vi "Dashboard Main.vi"() -> ()   [LabVIEW 2015]
uses:
  <vilib>/Utility/miscctls.llb/LVRowAndColumnTypeDef.ctl
  <vilib>/event_ctls.llb/eventvkey.ctl
  <vilib>/Rock Robotics/WPI/Dashboard/WPI_DashboardLogging Global.vi
  <vilib>/Rock Robotics/Network Tables/NT Read Numeric Array.vi
  <vilib>/Utility/config.llb/Write Key (String).vi
  <vilib>/Utility/config.llb/Write Key (I32).vi
  <vilib>/Utility/config.llb/NI_LVConfig.lvlib
panel:
  in  "Camera Settings 2":T1={"Frame Rate"=30, "Compression"=30, "Size"=1} {"Frame Rate" scale=1.0..30.0; "Size" items=["640x480", "320x240", "160x120"]}
  out "Camera IP 2":string
  in  "Rec Mode 2":enum32{"Stop", "Record", "Playback"}(radio)
  in  "Vision 2":u16(ring) items=["Camera Off", "USB Camera SW", "USB Camera HW", "IP Camera"]
  in  "TCP":refnum<k5>
  in  "Rec Mode":enum32{"Stop", "Record", "Playback"}(radio)
  in  "Vision":u16(ring) items=["Camera Off", "USB Camera SW", "USB Camera HW", "IP Camera"]
  out "Camera IP":string
  out "Image Message":string="Timeout in Camera Communications"
  in  "Dashboard Tab":T2(tab)
  in  "Select Auto":string(combo)
  out "NT Connection":bool
  in  "Camera Settings":T1={"Frame Rate"=30, "Compression"=30, "Size"=1} {"Frame Rate" scale=1.0..30.0; "Size" items=["640x480", "320x240", "160x120"]}
  out "MotorChart R":cluster{"Numeric":dbl, "Numeric":dbl}(graph)
  out "MotorChart L":T3(graph)
  out "MotorSliders R":cluster{"MotorSlide1":dbl, "MotorSlide2":dbl} {"MotorSlide2" scale=-1.0..1.0 scale format="%#_2e"; "MotorSlide1" scale=-1.0..1.0 scale format="%#_2e"}
  out "MotorSliders L":T4 {"MotorSlide4 2" scale=0.0..14.0 scale format="%#_2e"; "MotorSlide2" scale=-1.0..1.0 scale format="%#_2e"; "MotorSlide1" scale=-1.0..1.0 scale format="%#_2e"}
  out "JS1 Z":dbl(slide) scale=-1.0..1.0 scale format="%#_2e"
  out "JS1 Graph":cluster{"X":dbl, "Y":dbl}[](graph)
  out "JS1 Buttons":T5
  out "JS2 Z":dbl(slide) scale=-1.0..1.0 scale format="%#_2e"
  out "JS2 Graph":cluster{"X":dbl, "Y":dbl}[](graph)
  out "JS2 Buttons":T5
  out "Mode":T6(ring)=enum."Auto Disabled"
  in  "DB Camera Config":bool
  out "fps":dbl format="%#.1g"
  out "Mbps":dbl format="%#.1g"
  out "Mbps LED":bool
  out "Camera Image 2":T7(plugin-control)
  out "Mbps 2":dbl format="%#.1g"
  out "fps 2":dbl format="%#.1g"
  in  "DB/String 9":string
  in  "DB/String 8":string
  in  "DB/String 7":string
  in  "DB/String 6":string
  in  "DB/String 5":string
  in  "DB/String 4":string
  in  "DB/String 3":string
  in  "DB/String 2":string
  in  "DB/String 1":string
  in  "DB/String 0":string
  in  "DB/Slider 0":dbl(slide) scale=0.0..5.0
  in  "DB/Slider 1":dbl(slide) scale=0.0..5.0
  in  "DB/Slider 2":dbl(slide) scale=0.0..5.0
  in  "DB/Slider 3":dbl(slide) scale=0.0..5.0
  out "DB/LED 3":bool
  out "DB/LED 2":bool
  out "DB/LED 1":bool
  out "DB/LED 0":bool
  in  "DB/Button 3":bool
  in  "DB/Button 2":bool
  in  "DB/Button 1":bool
  in  "DB/Button 0":bool caption="New Name"
  in  "Test Slider":dbl(slide) scale=0.0..100.0 scale format="%#_3g"
  in  "On/Off":bool caption="Solenoid"
  in  "Test Name":u16(ring) items=["Select the test to run..."]
  in  "Test Tree":string(tree)
  in  "Motor":cluster{"Value":dbl, "Enable":bool} {"Value" scale=-1.0..1.0 scale format="%#_3g"}
  out "Progress":T8 {"Test Progress" scale=0.0..100.0}
  in  "Rev/Fwd":cluster{"Forward":bool, "Reverse":bool}
  in  "Test Ring":u16(ring) items=["Monochrome", "Color"]
  out "Cmd Status":string
  in  "Execute Command":bool
  in  "Command Params":string[][](table)
  in  "Command Selection":i32(listbox)
  in  "CheckList":i32(listbox)
  out "Tree":string(tree)
  out "Camera Image":T7(plugin-control)
  out "Background":bool
  # "Left"
  # "Front"
  # "Right"
  # "Battery"
  # "This tab is a great place for autonomous settings and robot-specific values.\nPlace controls and indicators inside this tab and match name to\nDashboard Variables on robot. You can also delete this comment."
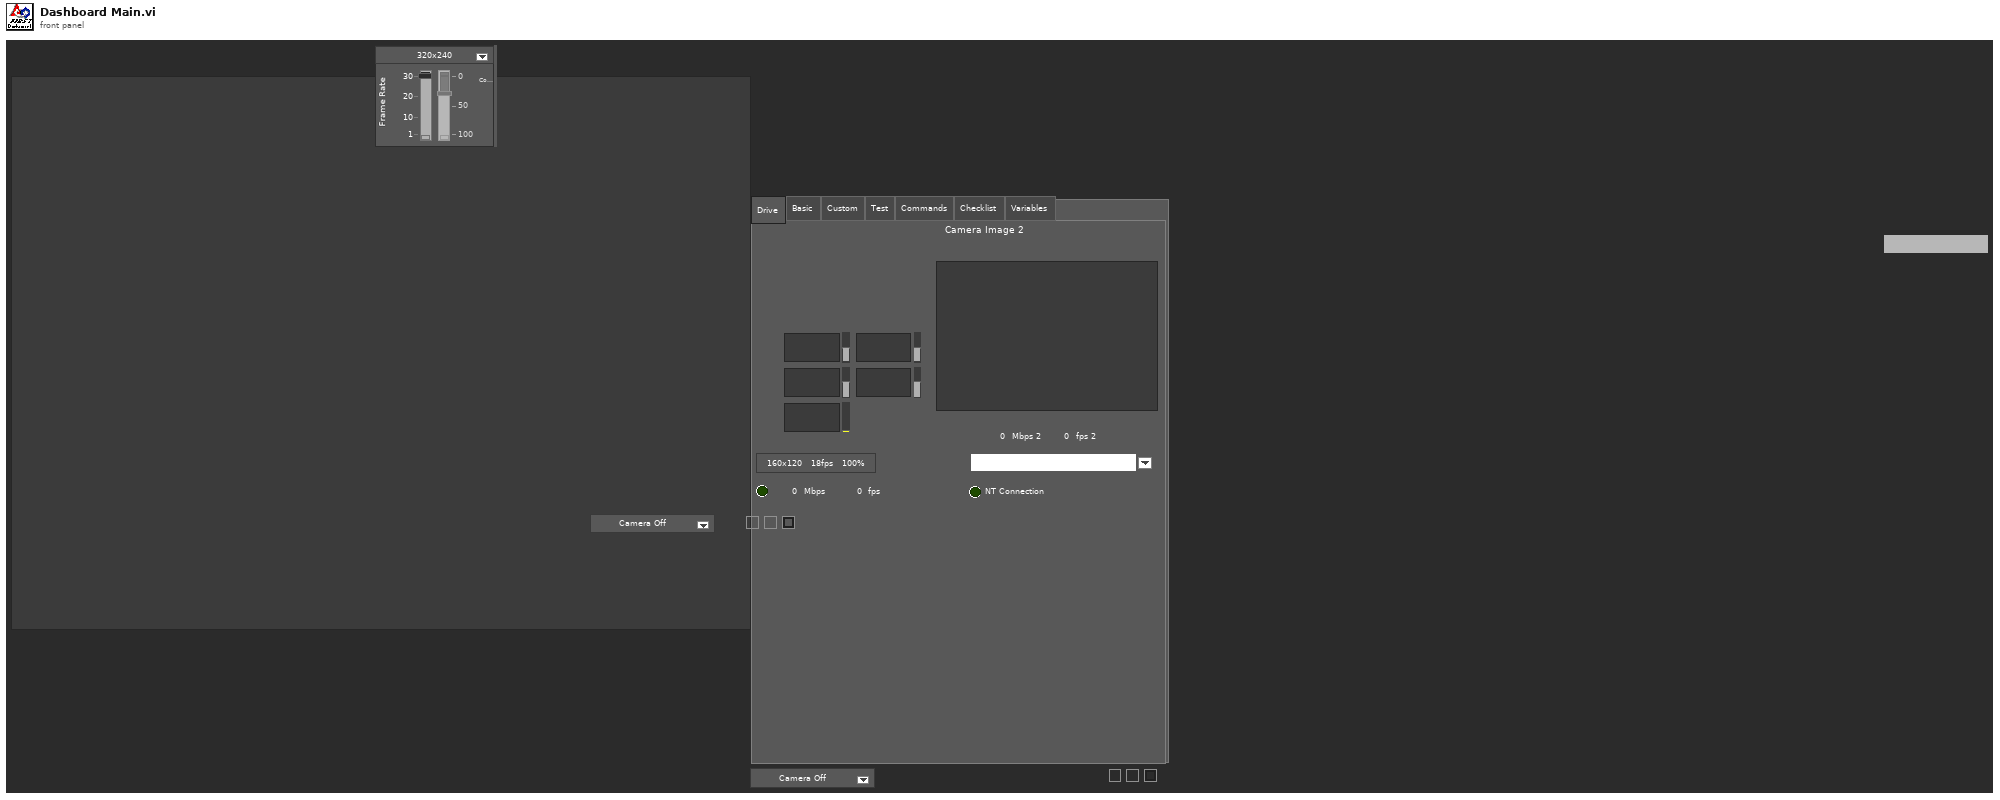
[diagram p1: front panel]
types:
  T1 = cluster{"Frame Rate":i32, "Compression":i32, "Size":u16}
  T2 = enum32{"Drive", "Basic", "Custom", "Test", "Commands", "Checklist", "Variables"}
  T3 = cluster{"Numeric":dbl, "Numeric":dbl, "Battery V":dbl}
  T4 = cluster{"MotorSlide1":dbl, "MotorSlide2":dbl, "MotorSlide4 2":dbl}
  T5 = cluster{bool, bool, bool, bool, bool, bool, bool, bool, bool, bool, bool, bool}
  T6 = enum8{"Tele-Op Disabled", "Tele-Op Enabled", "Auto Disabled", "Auto Enabled", "Test Disabled", "Test Enabled", "Disconnected", "No Code", "E-Stop"}
  T7 = typedef "IMAQ Image.ctl" = refnum<image>
  T8 = cluster{"Test Progress":u8, "Test Progress Text":string}
  T9 = typedef "Image Type" = u32
  T10 = cluster{"IDs":cluster{"RPC field ID":u16, "Unique ID":u16}, "String":string}
  T11 = enum32{"Drive", "Basic", "Custom", "Test", "Checklist", "Variables"}
  T12 = cluster{"Camera Image":refnum<vi>, "Dashboard Tab":refnum<vi>, "Background":refnum<vi>, "Vision":refnum<vi>, "Rec Mode":refnum<vi>, "Test Slider":refnum<vi>, "On/Off ":refnum<vi>, "Test Ring":refnum<vi>, "Rev/Fwd":refnum<vi>, "Test Name":refnum<vi>, "Motor":refnum<vi>, "Progress":refnum<vi>, "CheckList":refnum<vi>, "Tree":refnum<vi>, "Test Tree":refnum<vi>, "Command Params":refnum<vi>, "Command Selection":refnum<vi>, "Execute Command":refnum<vi>, "Cmd Status":refnum<vi>}
  T13 = cluster{"Error Strings":string, "Disable Counts":cluster{u16, u16}, "Rail Faults":cluster{u16, u16, u16}, "Robot IP":string, "DB Mode":u8, "Event Info":cluster{"Name":string, "Type":u8, "Number":u16, "Replay":u8}, "Camera Addr":string}
  T14 = cluster{"Storage":cluster{"Disk Free":u64, "RAM Block":u32, "RAM free":u32}, "CPU Utilization":cluster{"CPU % ISR":sgl, "CPU % Time Crit":sgl, "CPU % Timed Str":sgl, "CPU % High":sgl, "CPU % Above":sgl, "CPU % Normal":sgl, "CPU % Low":sgl}, "CAN":cluster{"% Bus Utilization":sgl, "Bus Off Cnt":u32, "TX_FIFO Full Cnt":u32, "Receive Error Cnt":u8, "Transmit Error Cnt":u8}, "HID":cluster{"HID Outputs":u32, "Rumble Low":u16, "Rumble High":u16}[]}
  T15 = cluster{"Status bits":cluster{"Test Mode":bool, "Autonomous":bool, "Enabled":bool, "Code Start":bool, "Brownout":bool, "Reserved 2":bool, "Reserved 3":bool, "E-Stop":bool}, "Code Trace":cluster{"Disabled":bool, "TeleOp":bool, "Auto":bool, "Test":bool}, "Controller Type":enum16{"unknown", "cRIO", "roboRio"}, "Code?":enum16{"unknown", "noCode", "code"}, "Battery V":dbl}
  T16 = cluster{"Control Bits":cluster{"TestMode":bool, "Autonomous":bool, "Enabled":bool, "FMS Present":bool, bool, bool, bool, "E-Stop":bool}, "Team Station ":u8, "Countdown":sgl, "Joystick Values":cluster{"Axes":dbl[], "Buttons":bool[], "POVs":i16[]}[]}
  T17 = cluster{"Axes":dbl[], "Buttons":bool[], "POVs":i16[]}[]
  T18 = cluster{"Axes":dbl[], "Buttons":bool[], "POVs":i16[]}
  T19 = cluster{"Buttons[0]":bool, "Buttons[1]":bool, "Buttons[2]":bool, "Buttons[3]":bool, "Buttons[4]":bool, "Buttons[5]":bool, "Buttons[6]":bool, "Buttons[7]":bool, "Buttons[8]":bool, "Buttons[9]":bool, "Buttons[10]":bool, "Buttons[11]":bool}
  T20 = typedef "NI_LVConfig.lvlib/Config Data RefNum.ctl" = refnum<k1>
  T21 = cluster{"Operation":enum16{"Update", "Clear"}, "Color Box":u32}[]
  T22 = typedef "eventvkey.ctl" = enum16{"ASCII", "Enter", "Return", "Shift", "Ctrl", "Alt", "Cmd", "Opt", "Caps", "NumLock", "Clear", "Break", "Up", "Down", "Left", "Right", "Insert", "Delete", "Home", "End", "PageUp", "PageDown", "Escape", "Help", "Pause", "ScrollLock", "F1", "F2", "F3", "F4", "F5", "F6", "F7", "F8", "F9", "F10", "F11", "F12", "F13", "F14", "F15", "F16", "F17", "F18", "F19", "F20", "F21", "F22", "F23", "F24", "Play", "VolumeUp", "VolumeDown", "Mute", "Two Byte Char"}
  T23 = cluster{"Image Size":bool, "Image Type":bool, "Pixel Value":bool, "ROI Information":bool, "Zoom Factor":bool}
  T24 = enum8{"Enabled", "Disabled", "Disabled and Grayed Out"}
  T25 = cluster{"Operation":enum16{"Update", "Clear"}, "Color Box":u32}
  T26 = typedef "LVRowAndColumnTypeDef.ctl" = cluster{"Row":i32, "Column":i32}
  T27 = cluster{"Shift":bool, "Ctrl":bool, "Alt":bool, "Cmd":bool, "Opt":bool}
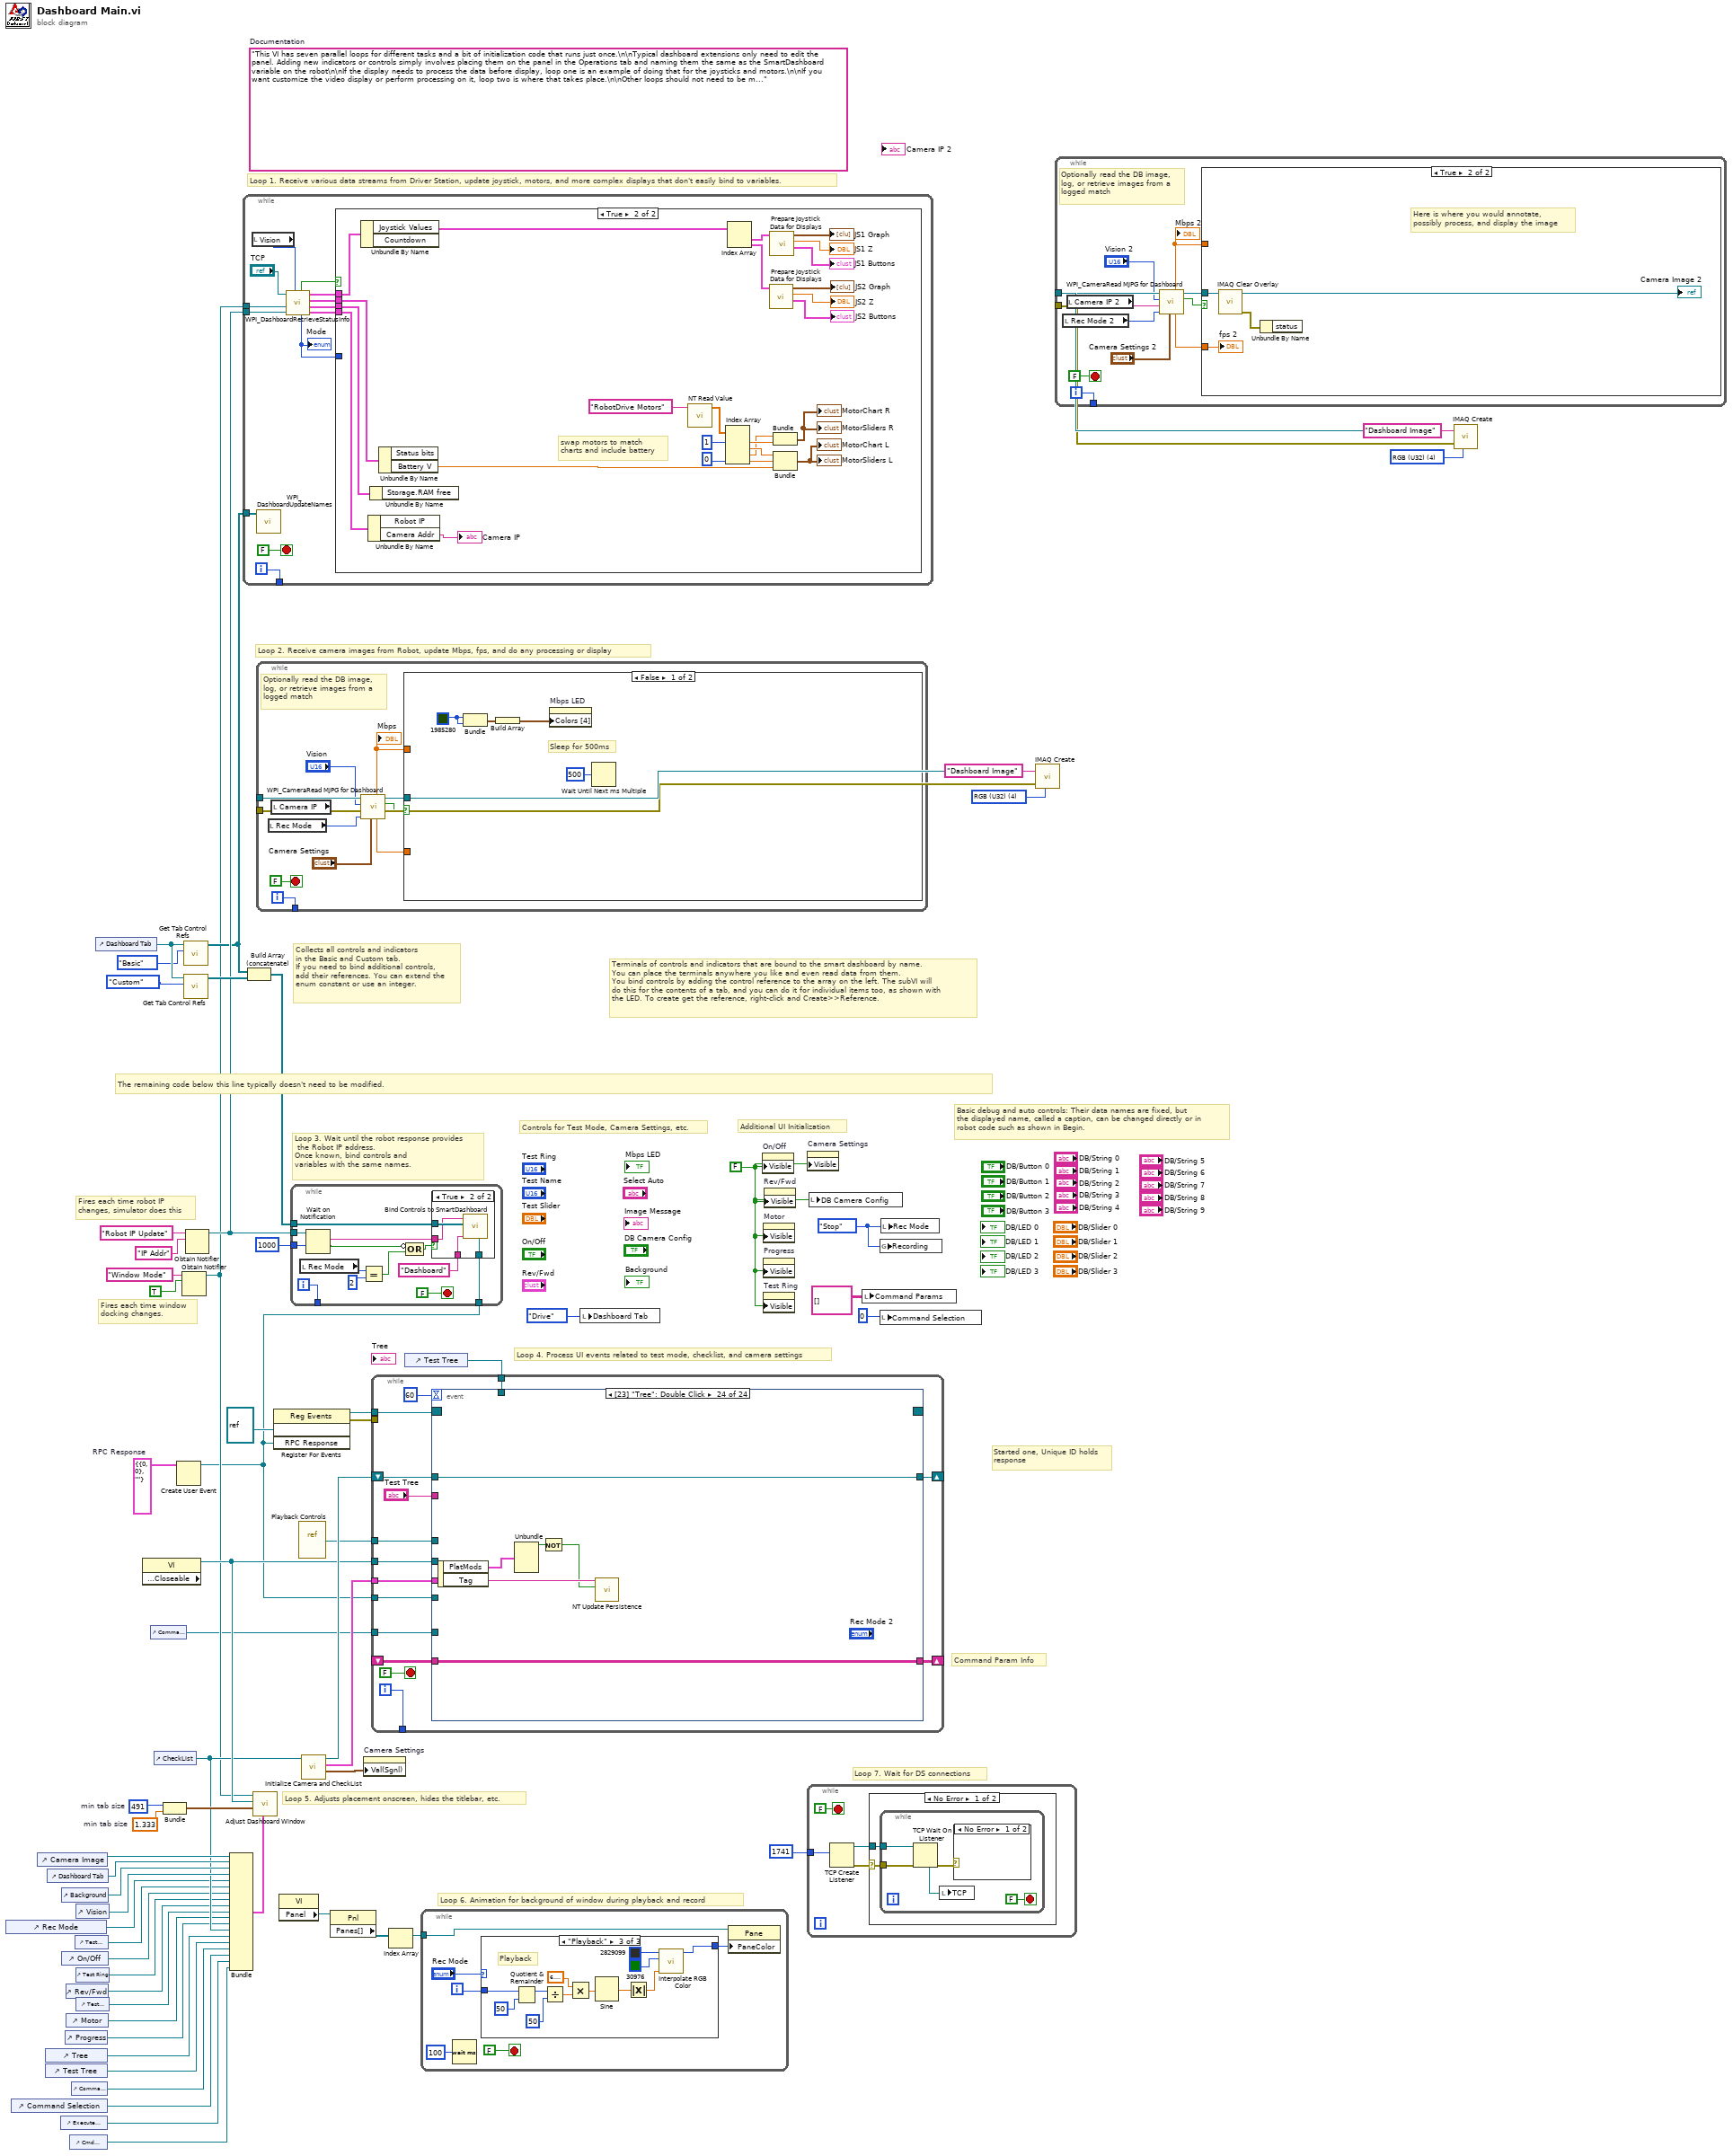
[diagram p0: block diagram]
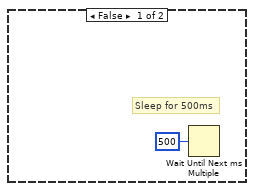
[diagram p2: hidden frame]
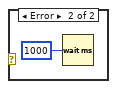
[diagram p3: hidden frame]
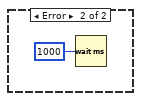
[diagram p4: hidden frame]
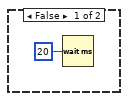
[diagram p5: hidden frame]
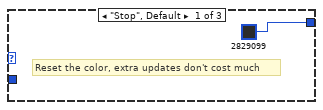
[diagram p6: hidden frame]
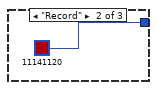
[diagram p7: hidden frame]
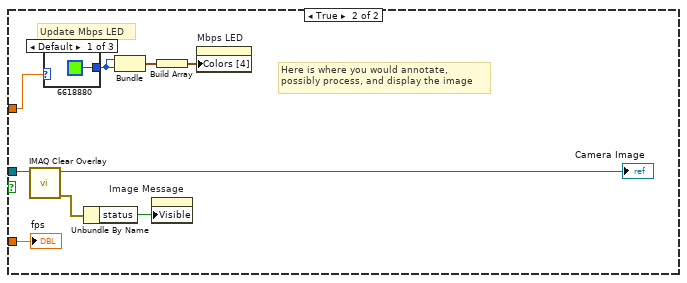
[diagram p9: hidden frame]
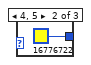
[diagram p10: hidden frame]
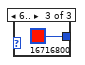
[diagram p11: hidden frame]
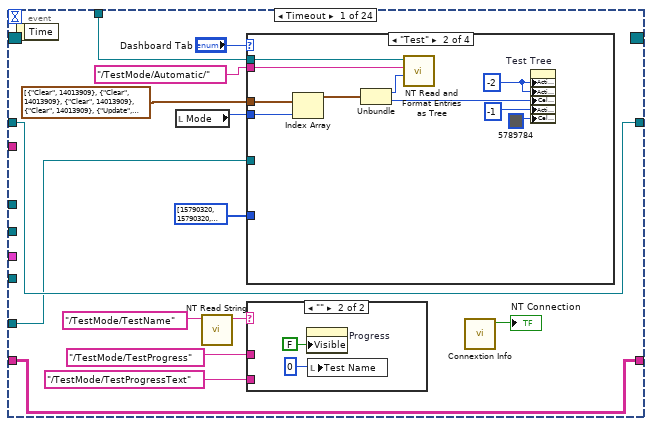
[diagram p12: hidden frame]
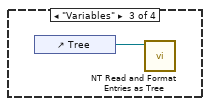
[diagram p14: hidden frame]
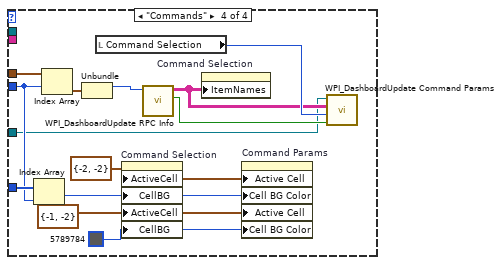
[diagram p15: hidden frame]
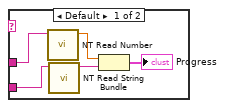
[diagram p16: hidden frame]
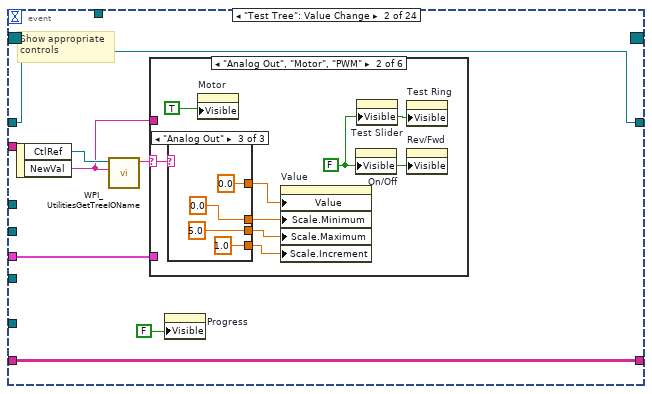
[diagram p17: hidden frame]
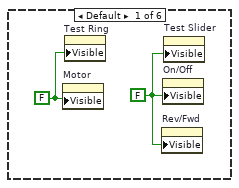
[diagram p18: hidden frame]
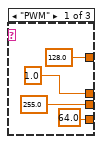
[diagram p19: hidden frame]
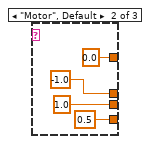
[diagram p20: hidden frame]
diagram:
  w4 = T9 4 items=["Grayscale (U8)", "Grayscale (I16)", "Grayscale (SGL)", "Complex (CSG)", "RGB (U32)", "HSL (U32)", "RGB (U64)"] ("Image Type")
  w11 = T10 {"IDs"={"RPC field ID"=0, "Unique ID"=0}, "String"=""}  # RPC Response
  w37 = 491  # min tab size
  w36 = 1.333  # min tab size
  w45 = enum32{"Stop", "Record", "Playback"}."Stop" ("Rec Mode")
  w19 = FALSE ("Visible")
  (unwired) "This VI has seven parallel loops for different tasks and a bit of initialization code that runs just once.\n\nTypical dashboard extensions only need to edit the panel. Adding new indicators or controls simply involves placing them on the panel in the Operations tab and naming them the same as the SmartDashboard variable on the robot\n\nIf the display needs to process the data before display, loop one is an example of doing that for the joysticks and motors.\n\nIf you want customize the video display or perform processing on it, loop two is where that takes place.\n\nOther loops should not need to be modified. They are pretty standard, and document the task they perform."  # Documentation
  w65 = T9 4 items=["Grayscale (U8)", "Grayscale (I16)", "Grayscale (SGL)", "Complex (CSG)", "RGB (U32)", "HSL (U32)", "RGB (U64)"] ("Image Type")
  # "Command Param Info"
  # "Started one, Unique ID holds\nresponse"
  # "Loop 7. Wait for DS connections"
  # "Basic debug and auto controls: Their data names are fixed, but\nthe displayed name, called a caption, can be changed directly or in\nrobot code such as shown in Begin."
  # "Controls for Test Mode, Camera Settings, etc."
  # "Additional UI Initialization"
  # "Loop 6. Animation for background of window during playback and record"
  # "Fires each time robot IP\nchanges, simulator does this"
  # "Fires each time window\ndocking changes."
  # "Collects all controls and indicators\nin the Basic and Custom tab.\nIf you need to bind additional controls,\nadd their references. You can extend the\nenum constant or use an integer."
  # "The remaining code below this line typically doesn't need to be modified."
  # "Loop 4. Process UI events related to test mode, checklist, and camera settings"
  # "Terminals of controls and indicators that are bound to the smart dashboard by name.\nYou can place the terminals anywhere you like and even read data from them.\nYou bind controls by adding the control reference to the array on the left. The subVI will\ndo this for the contents of a tab, and you can do it for individual items too, as shown with\nthe LED. To create get the reference, right-click and Create>>Reference."
  # "Loop 3. Wait until the robot response provides\n the Robot IP address.\nOnce known, bind controls and\nvariables with the same names."
  # "Loop 5. Adjusts placement onscreen, hides the titlebar, etc."
  # "Loop 1. Receive various data streams from Driver Station, update joystick, motors, and more complex displays that don't easily bind to variables."
  # "Loop 2. Receive camera images from Robot, update Mbps, fps, and do any processing or display"
  n1 = control-ref of="Rec Mode"() -> (w25:refnum<vi>)
  n2 = control-ref of="Command Selection"() -> (w10:refnum<vi>)
  n3 = control-ref of="Camera Image"() -> (w40:refnum<vi>)
  n4 = control-ref of="Tree"() -> (w29:refnum<vi>)
  n5 = control-ref of="Test Tree"() -> (w28:refnum<vi>)
  n6 = control-ref of="Dashboard Tab"() -> (w39:refnum<vi>)
  n7 = control-ref of="Execute Command"() -> (w12:refnum<vi>)
  n8 = control-ref of="Background"() -> (w34:refnum<vi>)
  n9 = control-ref of="On/Off"() -> (w23:refnum<vi>)
  n10 = control-ref of="Progress"() -> (w20:refnum<vi>)
  n11 = control-ref of="Rev/Fwd"() -> (w21:refnum<vi>)
  n12 = control-ref of="Motor"() -> (w26:refnum<vi>)
  n13 = control-ref of="Cmd Status"() -> (w6:refnum<vi>)
  n14 = control-ref of="Command Params"() -> (w13:refnum<vi>)
  n15 = control-ref of="Test Slider"() -> (w24:refnum<vi>)
  n16 = control-ref of="Vision"() -> (w38:refnum<vi>)
  n17 = control-ref of="Test Ring"() -> (w22:refnum<vi>)
  n18 = control-ref of="Test Name"() -> (w27:refnum<vi>)
  n19 = control-ref of="Dashboard Tab"() -> (w43:refnum<vi>)
  n20 = property class="VI" props=["Front Panel.Closeable"]() -> (reference out=w44:refnum<vi>)  [unwired: 2 in, 2 out]
  n21 = control-ref of="Command Params"() -> (w5:refnum<vi>)
  n22 = control-ref of="CheckList"() -> (w30:refnum<vi>)
  n23 = Bundle("min tab size"=w37, "min tab size"=w36) -> (w35:cluster{"min tab size":i32, "min tab size":dbl})  [unwired: 1 in]
  n24 = Create User Event(user event datatype=w11) -> (user event=w7:refnum<user-event>)  [unwired: 1 in, 1 out]
  n25 = Obtain Notifier(name (unnamed)="Window Mode", notification data type=TRUE) -> (notifier out=w16:refnum<notifier>)  [unwired: 2 in, 2 out]
  n26 = call <vilib>:"Get Tab Control Refs.vi"("Page Index"=T11."Basic" ("Dashboard Tab"), "TabControl in"=w43) -> ("ControlsOnPage"=w17:refnum<vi>[])  [unwired: 9 in]
  n27 = call <vilib>:"Get Tab Control Refs.vi"("Page Index"=T11."Custom" ("Dashboard Tab"), "TabControl in"=w43) -> ("ControlsOnPage"=w42:refnum<vi>[])  [unwired: 9 in]
  n28 = Obtain Notifier(name (unnamed)="Robot IP Update", notification data type="IP Addr" ("name (unnamed)")) -> (notifier out=w18:refnum<notifier>)  [unwired: 2 in, 2 out]
  n29 = Bundle("Camera Image"=w40, "Dashboard Tab"=w39, "Background"=w34, "Vision"=w38, "Rec Mode"=w25, "Test Slider"=w24, "On/Off"=w23, "Test Ring"=w22, "Rev/Fwd"=w21, "Test Name"=w27, "Motor"=w26, "Progress"=w20, "CheckList"=w30, "Tree"=w29, "Test Tree"=w28, "Command Params"=w13, "Command Selection"=w10, "Execute Command"=w12, "Cmd Status"=w6) -> (w31:T12)  [unwired: 1 in]
  n30 = while {
    tunnel: [w77] -> _
    tunnel: w18 -> [w71]
    tunnel: w17 -> [w70]
    tunnel: w16 -> [w66]
    i -> [w77]
    stop <- FALSE stop-if-true
    n31 = local read "Vision"() -> (w68:u16)
    n32 = call <vilib>:"WPI_DashboardUpdateNames.vi"("Controls on Tab"=w70) -> ()  [unwired: 11 in]
    n33 = call <vilib>:"WPI_DashboardRetrieveStatusInfo.vi"("Vision"=w68, "Binding Refnum"=w71, "Window Mode Notifier"=w66, "TCP Cnx"="TCP") -> ("Power and Errors"=w72:T13, "Robot Metrics"=w75:T14, "Status Info"=w76:T15, "Control Info"=w73:T16, "Robot Mode"=w69:T6, "Process?"=w74:bool)  [unwired: 2 in]
    "Mode" <- w69
    n34 = case shown="True" w74 {
      tunnel: w76 -> [_ w104]
      tunnel: w75 -> [_ w103]
      tunnel: w73 -> [_ w102]
      tunnel: w72 -> [_ w101]
      tunnel: w69 -> [_ _]
      frame False {
        n35 = Wait (ms)(milliseconds to wait=u32 20) -> ()  [unwired: 1 out]
      }
      frame True {
        # "swap motors to match\ncharts and include battery"
        n36 = Unbundle By Name(w102) -> ("Joystick Values"=w91:T17)  [unwired: 1 out]
        n37 = Unbundle By Name(w101) -> ("Camera Addr"=→"Camera IP":string)  [unwired: 1 out]
        n38 = Unbundle By Name(w103) -> ()  [unwired: 1 out]
        n39 = Unbundle By Name(w104) -> ("Battery V"=w92:dbl)  [unwired: 1 out]
        n40 = call-poly <vilib>:"NT Read Value.vi"("Name"="RobotDrive Motors") -> ("Numeric Array"=w80:dbl[])  [unwired: 9 in, 1 out]
        n41 = Index Array(array=w80, index #1=1, index #4=0) -> (element #1=w96:dbl, element #2=w97:dbl, element #3=w95:dbl, element #4=w100:dbl)  [unwired: 2 in]
        n42 = Index Array(array=w91) -> (element #1=w90:T18, element #2=w85:T18)  [unwired: 2 in]
        n43 = call "Prepare Joystick Data for Displays.vi"("Joystick Values"=w85) -> ("Buttons"=→"JS2 Buttons":T19, "Z Axis"=→"JS2 Z":dbl, "Cartesian Data"=→"JS2 Graph":cluster{"X axis":dbl, "X axis":dbl}[])  [unwired: 8 in]
        n44 = call "Prepare Joystick Data for Displays.vi"("Joystick Values"=w90) -> ("Buttons"=→"JS1 Buttons":T19, "Z Axis"=→"JS1 Z":dbl, "Cartesian Data"=→"JS1 Graph":cluster{"X axis":dbl, "X axis":dbl}[])  [unwired: 8 in]
        n45 = Bundle("Numeric"=w95, "Numeric"=w96) -> (→"MotorChart R" →"MotorSliders R":cluster{"Numeric":dbl, "Numeric":dbl})  [unwired: 1 in]
        n46 = Bundle("Numeric"=w97, "Numeric"=w100, "Battery V"=w92) -> (→"MotorChart L" →"MotorSliders L":T3)  [unwired: 1 in]
      }
    }
  }
  n47 = Build Array (concatenate)(w17, w42) -> (w41:refnum<vi>[])
  n48 = call "Adjust Dashboard Window.vi"("Sizing Refnums"=w31, "Size Constraints"=w35, "VI"=w44, "WIn Mode"=w16) -> ()  [unwired: 8 in]
  n49 = register-events(refnum<vi> refnum, w7) -> (reference out=w49:refnum<event-registration>, error out=w48:errorcluster)  [unwired: 2 in]
  n50 = property class="VI"() -> ("Panel"=w52:refnum<vi>)  [unwired: 2 in, 2 out]
  n51 = while {
    tunnel: w41 -> [w117]
    tunnel: w18 -> [w115]
    tunnel: [w113] -> _
    tunnel: u32 1000 ("milliseconds to wait") -> [w112]
    tunnel: w7 -> [w105]
    i -> [w113]
    stop <- FALSE stop-if-true
    n52 = local read "Rec Mode"() -> (w108:enum32{"Stop", "Record", "Playback"})
    n53 = Wait on Notification(notifier=w115, timeout in ms (-1)=w112) -> (notification=w114:string, timed out?=w110:bool)  [unwired: 2 in, 2 out]
    n54 = Equal?(x=w108, y=u16 2 ("Rec Mode")) -> (x = y?=w109:bool)
    n55 = Compound Arithmetic op=OR(invert w110, w109) -> (w111:bool)
    n56 = case shown="True" w111 {
      tunnel: w117 -> [_ w121]
      tunnel: w114 -> [_ w120]
      tunnel: "Dashboard" -> [_ w119]
      tunnel: w105 -> [_ w118]
      frame False {
      }
      frame True {
        n57 = call <vilib>:"Bind Controls to SmartDashboard.vi"("RPC ref"=w118, "Client Name"=w119, "Bound Control Refs"=w121, "Server IP Address"=w120) -> ()  [unwired: 8 in]
      }
    }
  }
  n58 = vi-ref "Playback Controls.vi"() -> (w50:refnum<vi>)
  n59 = call "Initialize Camera and CheckList.vi"("ListBox in"=w30) -> ("Cluster"=w56:cluster{"value":i32, "value":i32, "index":i32}, "Array"=w57:cluster{string[]}[], "File Refnum"=w55:T20)  [unwired: 8 in]
  n60 = property class="Pnl"(reference=w52) -> ("Panes[]"=w53:refnum<vi>[])  [unwired: 1 in, 2 out]
  n61 = property on="Camera Settings" class="Clust (strict)"("Val(Sgnl)"=w56) -> ()  [unwired: 2 in, 2 out]
  n62 = Index Array(array=w53) -> (element=w51:refnum<vi>)  [unwired: 1 in]
  n63 = control-ref of="Test Tree"() -> (w54:refnum<vi>)
  n64 = while {
    tunnel: w57 -> [w133]
    shift-right: [w132] -> _
    shift-left: w55 -> [w131]
    tunnel: [w130] -> _
    tunnel: w54 -> [w129]
    tunnel: w50 -> [w128]
    tunnel: w49 -> [w127]
    tunnel: w48 -> [_]
    tunnel: w44 -> [w126]
    tunnel: w7 -> [w125]
    tunnel: w5 -> [w124]
    shift-right: [w123] -> _
    shift-left: _ -> [w122]
    i -> [w130]
    stop <- FALSE stop-if-true
    n65 = event shown="[23] \"Tree\": Double Click" {
      selector: w127 -> [_ _ _ _ _ _ _ _ _ _ _ _ _ _ _ _ _ _ _ _ _ _ _ _]
      dyn-events: [_ _ _ _ _ _ _ _ _ _ _ _ _ _ _ _ _ _ w442 _ _ _ _ _] -> _
      timeout: u32 60 ("milliseconds to wait") -> [_ _ _ _ _ _ _ _ _ _ _ _ _ _ _ _ _ _ _ _ _ _ _ _]
      tunnel: w129 -> [w146 _ _ _ _ _ _ _ _ _ _ _ _ _ _ _ _ _ _ _ _ _ _ _]
      tunnel: "Test Tree" -> [_ _ _ _ _ _ _ _ _ _ _ _ _ w405 w414 w417 w422 w431 _ _ _ _ _ _]
      tunnel: w133 -> [_ w184 _ _ _ _ _ _ _ _ _ w367 w398 _ _ _ _ _ _ _ _ _ _ _]
      tunnel: [w143 w183 w287 w293 w303 w307 w313 w325 w333 w339 w352 w366 w391 w404 w412 w416 w421 w430 w444 w460 w462 w470 w481 w486] -> w132
      tunnel: w131 -> [w143 w183 w287 w293 w303 w307 w313 w325 w333 w339 w352 w365 w391 w404 w412 w416 w421 w430 w444 w460 w462 w470 w481 w486]
      tunnel: w128 -> [_ _ _ _ _ _ _ _ _ _ _ _ _ _ _ _ _ _ w445 _ w465 _ _ _]
      tunnel: w126 -> [_ _ _ _ _ _ _ _ _ _ _ _ _ _ _ _ _ _ w440 _ _ _ _ _]
      tunnel: w125 -> [_ _ _ _ _ _ _ _ _ _ _ _ _ _ _ _ _ _ w436 _ _ _ _ _]
      tunnel: w124 -> [w138 _ _ _ _ _ w311 _ _ _ _ _ _ _ _ _ _ _ _ _ _ _ _ _]
      tunnel: [w137 w182 w286 w292 w302 w308 w309 w319 w330 w338 w351 w364 w390 w403 w411 w415 w420 w429 w435 w458 w461 w466 w474 w487] -> w123
      tunnel: w122 -> [w137 w182 w286 w292 w302 w308 w309 _ _ w338 w351 w364 w390 w403 w411 w415 w420 w429 w435 w458 w461 w466 w474 w487]
      event Timeout {
        n66 = event-data() -> ()  [unwired: 1 in, 1 out]
        n67 = local read "Mode"() -> (w140:T6)
        n68 = call <vilib>:"NT Read String.vi"("Name"="/TestMode/TestName") -> ("String"=w149:string)  [unwired: 9 in, 1 out]
        n69 = case shown="\"Test\"" "Dashboard Tab" {
          tunnel: w146 -> [_ w160 _ _]
          tunnel: "/TestMode/Automatic/" ("Name Pattern") -> [_ w159 _ _]
          tunnel: T21 [{"Operation"=enum."Clear", "Color Box"=14013909}, {"Operation"=enum."Clear", "Color Box"=14013909}, {"Operation"=enum."Clear", "Color Box"=14013909}, {"Operation"=enum."Clear", "Color Box"=14013909}, {"Operation"=enum."Update", "Color Box"=14013909}, {"Operation"=enum."Update", "Color Box"=16777215}, {"Operation"=enum."Clear", "Color Box"=14013909}, {"Operation"=enum."Clear", "Color Box"=14013909}, {"Operation"=enum."Clear", "Color Box"=14013909}] -> [_ w152 _ w169]
          tunnel: w140 -> [_ w151 _ w168]
          tunnel: u32[] [15790320, 15790320, 15790320, 15790320, 16777215, 16777215, 15790320, 15790320, 15790320] -> [_ _ _ w174]
          tunnel: w138 -> [_ _ _ w162]
          frame "Custom", Default {
          }
          frame "Test" {
            w158 = -2 ("Active Item:Row Number")
            n70 = Index Array(array=w152, index=w151) -> (element=w153:T25)
            n71 = Unbundle(w153) -> ("Operation"=w154:enum16{"Update", "Clear"}, "Color Box"=w155:u32)
            n72 = call <vilib>:"NT Read and Format Entries as Tree.vi"("Operation"=w154, "Name Pattern"=w159, "Tree Refnum"=w160) -> ()  [unwired: 7 in, 2 out]
            n73 = property on="Test Tree" class="Tree (strict)"("Active Item Row Number"=w158, "ActiveColNum"=w158, "CellBG"=w155, "Active Item Row Number"=-1 ("Active Item:Row Number"), "CellBG"=u32 5789784 ("Color Box")) -> ()  [unwired: 2 in, 2 out]
          }
          frame "Variables" {
            n74 = control-ref of="Tree"() -> (w161:refnum<vi>)
            n75 = call <vilib>:"NT Read and Format Entries as Tree.vi"("Tree Refnum"=w161) -> ()  [unwired: 9 in, 2 out]
          }
          frame "Commands" {
            w170 = u32 5789784 ("Color Box")
            w171 = T26 {"Row"=-1, "Column"=-2} ("Active Cell:Active Cell")
            w173 = T26 {"Row"=-2, "Column"=-2} ("Active Cell:Active Cell")
            n76 = Index Array(array=w174, index=w168) -> (element=w172:u32)
            n77 = Index Array(array=w169, index=w168) -> (element=w167:T25)
            n78 = Unbundle(w167) -> ("Operation"=w166:enum16{"Update", "Clear"})  [unwired: 1 out]
            n79 = local read "Command Selection"() -> (w165:i32)
            n80 = property on="Command Selection" class="MCListbox (strict)"("ActiveCell"=w173, "CellBG"=w172, "ActiveCell"=w171, "CellBG"=w170) -> ()  [unwired: 2 in, 2 out]
            n81 = call <vilib>:"WPI_DashboardUpdate RPC Info.vi"("Operation"=w166) -> ("update"=w164:bool, "commands"=w163:string[][])  [unwired: 9 in]
            n82 = property on="Command Selection" class="MCListbox (strict)"("ItemNames"=w163) -> ()  [unwired: 2 in, 2 out]
            n83 = property on="Command Params" class="Tbl (strict)"("Active Cell"=w173, "Cell BG Color"=w172, "Active Cell"=w171, "Cell BG Color"=w170) -> ()  [unwired: 2 in, 2 out]
            n84 = call <vilib>:"WPI_DashboardUpdate Command Params.vi"("Update"=w164, "NewVal"=w165, "Commands"=w163, "Param Tbl"=w162) -> ()  [unwired: 7 in, 1 out]
          }
        }
        n85 = case shown="\"\"" w149 {
          tunnel: "/TestMode/TestProgress" ("Name") -> [w176 _]
          tunnel: "/TestMode/TestProgressText" ("Name") -> [w175 _]
          frame Default {
            n86 = call <vilib>:"NT Read Number.vi"("Name"=w176) -> ("Numeric"=w177:dbl)  [unwired: 9 in, 1 out]
            n87 = call <vilib>:"NT Read String.vi"("Name"=w175) -> ("String"=w178:string)  [unwired: 9 in, 1 out]
            n88 = Bundle("Numeric"=w177, "String"=w178) -> (→"Progress":cluster{"Numeric":dbl, "String":string})  [unwired: 1 in]
          }
          frame "" {
            n89 = property on="Progress" class="Clust (strict)"("Visible"=FALSE) -> ()  [unwired: 2 in, 2 out]
            n90 = local write "Test Name"(u16 0) -> ()
          }
        }
        n91 = call <vilib>:"Connextion Info.vi"() -> ("Connected"=→"NT Connection":bool)  [unwired: 10 in, 1 out]
      }
      event "Test Tree": Value Change {
        # "Show appropriate\ncontrols"
        n92 = event-data() -> ("CtlRef"=w187:refnum<vi>, "NewVal"=w185:string)  [unwired: 1 in]
        n93 = call <vilib>:"WPI_UtilitiesGetTreeIOName.vi"("NewVal"=w185, "TreeControl in"=w187) -> ("I/O Name"=w188:string)  [unwired: 9 in]
        n94 = case shown="\"Analog Out\", \"Motor\", \"PWM\"" w188 {
          selector: w188 -> [_ w195 _ w217 w226 _]
          tunnel: w185 -> [_ _ w214 w216 _ w233]
          tunnel: w184 -> [_ _ _ _ _ w232]
          frame Default {
            w190 = FALSE ("Visible")
            w189 = FALSE ("Visible")
            n95 = property on="Motor" class="Clust (strict)"("Visible"=w189) -> ()  [unwired: 2 in, 2 out]
            n96 = property on="Test Ring" class="Ring (strict)"("Visible"=w189) -> ()  [unwired: 2 in, 2 out]
            n97 = property on="Rev/Fwd" class="Clust (strict)"("Visible"=w190) -> ()  [unwired: 2 in, 2 out]
            n98 = property on="On/Off" class="Bool (strict)"("Visible"=w190) -> ()  [unwired: 2 in, 2 out]
            n99 = property on="Test Slider" class="Slide (strict)"("Visible"=w190) -> ()  [unwired: 2 in, 2 out]
          }
          frame "Analog Out", "Motor", "PWM" {
            w196 = FALSE ("Visible")
            n100 = case shown="\"Analog Out\"" w195 {
              tunnel: [1.0 ("Value") -1.0 ("Value") 0.0 ("Value")] -> w194
              tunnel: [255.0 ("Value") 1.0 ("Value") 5.0 ("Value")] -> w193
              tunnel: [128.0 ("Value") 0.0 ("Value") 0.0 ("Value")] -> w192
              tunnel: [64.0 ("Value") 0.5 ("Value") 1.0 ("Value")] -> w191
              frame "PWM" {
              }
              frame "Motor", Default {
              }
              frame "Analog Out" {
              }
            }
            n101 = property on="Motor" class="Clust (strict)"("Visible"=TRUE) -> ()  [unwired: 2 in, 2 out]
            n102 = property on="Value" class="Slide (strict)"("Value"=w192, "Scale.Minimum"=w194, "Scale.Maximum"=w193, "Scale.Increment"=w191) -> ()  [unwired: 2 in, 2 out]
            n103 = property on="On/Off" class="Bool (strict)"("Visible"=w196) -> ()  [unwired: 2 in, 2 out]
            n104 = property on="Test Slider" class="Slide (strict)"("Visible"=w196) -> ()  [unwired: 2 in, 2 out]
            n105 = property on="Test Ring" class="Ring (strict)"("Visible"=w196) -> ()  [unwired: 2 in, 2 out]
            n106 = property on="Rev/Fwd" class="Clust (strict)"("Visible"=w196) -> ()  [unwired: 2 in, 2 out]
          }
          frame "Servo" {
            w212 = FALSE ("Visible")
            n107 = call <vilib>:"NT Read Number.vi"("Name"=w214) -> ("Numeric"=w213:dbl)  [unwired: 9 in, 1 out]
            n108 = property on="Test Slider" class="Slide (strict)"("Visible"=TRUE, "Scale.Maximum"=170.0 ("Scale.Range:Maximum")) -> ()  [unwired: 2 in, 2 out]
            n109 = local write "Test Slider"(w213) -> ()
            n110 = property on="Motor" class="Clust (strict)"("Visible"=w212) -> ()  [unwired: 2 in, 2 out]
            n111 = property on="Rev/Fwd" class="Clust (strict)"("Visible"=w212) -> ()  [unwired: 2 in, 2 out]
            n112 = property on="On/Off" class="Bool (strict)"("Visible"=w212) -> ()  [unwired: 2 in, 2 out]
            n113 = property on="Test Ring" class="Ring (strict)"("Visible"=w212) -> ()  [unwired: 2 in, 2 out]
          }
          frame "Relay", "Solenoid" {
            w215 = FALSE ("Visible")
            n114 = property on="Motor" class="Clust (strict)"("Visible"=w215) -> ()  [unwired: 2 in, 2 out]
            n115 = property on="Test Slider" class="Slide (strict)"("Visible"=w215) -> ()  [unwired: 2 in, 2 out]
            n116 = Search and Replace String(input string=w216, search string="/Value  **", replace string="/Direction") -> (result string=w222:string)  [unwired: 5 in, 3 out]
            n117 = property on="Test Ring" class="Ring (strict)"("Visible"=w215) -> ()  [unwired: 2 in, 2 out]
            n118 = call <vilib>:"NT Read String.vi"("Name"=w222) -> ("String"=w220:string)  [unwired: 9 in, 1 out]
            n119 = Equal?(x="Both directions", y=w220) -> (x = y?=w218:bool)
            n120 = Not(x=w218) -> (.not. x?=w219:bool)
            n121 = property on="Rev/Fwd" class="Clust (strict)"("Visible"=w218) -> ()  [unwired: 2 in, 2 out]
            n122 = property on="On/Off" class="Bool (strict)"("Visible"=w219, "Caption.Text"=w217) -> ()  [unwired: 2 in, 2 out]
          }
          frame "Compressor", "Digital Out" {
            w225 = FALSE ("Visible")
            # "Get direction and finish"
            n123 = property on="Motor" class="Clust (strict)"("Visible"=w225) -> ()  [unwired: 2 in, 2 out]
            n124 = property on="Test Slider" class="Slide (strict)"("Visible"=w225) -> ()  [unwired: 2 in, 2 out]
            n125 = property on="Test Ring" class="Ring (strict)"("Visible"=w225) -> ()  [unwired: 2 in, 2 out]
            n126 = property on="On/Off" class="Bool (strict)"("Visible"=TRUE, "Caption.Text"=w226) -> ()  [unwired: 2 in, 2 out]
            n127 = property on="Rev/Fwd" class="Clust (strict)"("Visible"=FALSE) -> ()  [unwired: 2 in, 2 out]
          }
          frame "Camera" {
            n128 = call <vilib>:"Get Last Path Segment.vi"("String in"=w233) -> ("String out"=w234:string)  [unwired: 10 in]
            n129 = property on="On/Off" class="Bool (strict)"("Visible"=FALSE) -> ()  [unwired: 2 in, 2 out]
            n130 = property on="Motor" class="Clust (strict)"("Visible"=FALSE) -> ()  [unwired: 2 in, 2 out]
            n131 = property on="Rev/Fwd" class="Clust (strict)"("Visible"=FALSE) -> ()  [unwired: 2 in, 2 out]
            n132 = case shown="\"White Balance  **\"" w234 {
              tunnel: w233 -> [w240 w249 w258 w267 w276 _ w282]
              tunnel: w232 -> [w238 w246 w255 w264 w273 _ _]
              frame "Size  **" {
                n133 = Index Array(array=w238) -> (element=w237:cluster{string[]})  [unwired: 1 in]
                n134 = call <vilib>:"NT Read String.vi"("Name"=w240) -> ("String"=w239:string)  [unwired: 9 in, 1 out]
                n135 = Unbundle(w237) -> (w235:string[])
                n136 = Match First String(2:w235, 3:w239) -> (0:w236:i32)  [unwired: 1 out]
                n137 = property on="Test Ring" class="Ring (strict)"("Value"=w236, "Strings []"=w235) -> ()  [unwired: 2 in, 2 out]
                n138 = property on="Test Ring" class="Ring (strict)"("Visible"=TRUE) -> ()  [unwired: 2 in, 2 out]
                n139 = property on="Test Slider" class="Slide (strict)"("Visible"=FALSE) -> ()  [unwired: 2 in, 2 out]
              }
              frame "White Balance  **" {
                n140 = Index Array(array=w246, index=1) -> (element=w247:cluster{string[]})
                n141 = call <vilib>:"NT Read String.vi"("Name"=w249) -> ("String"=w248:string)  [unwired: 9 in, 1 out]
                n142 = Unbundle(w247) -> (w244:string[])
                n143 = Match First String(2:w244, 3:w248) -> (0:w243:i32)  [unwired: 1 out]
                n144 = property on="Test Ring" class="Ring (strict)"("Value"=w243, "Strings []"=w244) -> ()  [unwired: 2 in, 2 out]
                n145 = property on="Test Ring" class="Ring (strict)"("Visible"=TRUE) -> ()  [unwired: 2 in, 2 out]
                n146 = property on="Test Slider" class="Slide (strict)"("Visible"=FALSE) -> ()  [unwired: 2 in, 2 out]
              }
              frame "Exposure  **" {
                n147 = Index Array(array=w255, index=2) -> (element=w256:cluster{string[]})
                n148 = call <vilib>:"NT Read String.vi"("Name"=w258) -> ("String"=w257:string)  [unwired: 9 in, 1 out]
                n149 = Unbundle(w256) -> (w252:string[])
                n150 = Match First String(2:w252, 3:w257) -> (0:w253:i32)  [unwired: 1 out]
                n151 = property on="Test Ring" class="Ring (strict)"("Value"=w253, "Strings []"=w252) -> ()  [unwired: 2 in, 2 out]
                n152 = property on="Test Ring" class="Ring (strict)"("Visible"=TRUE) -> ()  [unwired: 2 in, 2 out]
                n153 = property on="Test Slider" class="Slide (strict)"("Visible"=FALSE) -> ()  [unwired: 2 in, 2 out]
              }
              frame "Exposure Priority  **" {
                n154 = Index Array(array=w264, index=3) -> (element=w265:cluster{string[]})
                n155 = call <vilib>:"NT Read String.vi"("Name"=w267) -> ("String"=w266:string)  [unwired: 9 in, 1 out]
                n156 = Unbundle(w265) -> (w261:string[])
                n157 = Match First String(2:w261, 3:w266) -> (0:w262:i32)  [unwired: 1 out]
                n158 = property on="Test Ring" class="Ring (strict)"("Value"=w262, "Strings []"=w261) -> ()  [unwired: 2 in, 2 out]
                n159 = property on="Test Ring" class="Ring (strict)"("Visible"=TRUE) -> ()  [unwired: 2 in, 2 out]
                n160 = property on="Test Slider" class="Slide (strict)"("Visible"=FALSE) -> ()  [unwired: 2 in, 2 out]
              }
              frame "Color Enable  **" {
                n161 = Index Array(array=w273, index=4) -> (element=w274:cluster{string[]})
                n162 = call <vilib>:"NT Read String.vi"("Name"=w276) -> ("String"=w275:string)  [unwired: 9 in, 1 out]
                n163 = Unbundle(w274) -> (w270:string[])
                n164 = Match First String(2:w270, 3:w275) -> (0:w271:i32)  [unwired: 1 out]
                n165 = property on="Test Ring" class="Ring (strict)"("Value"=w271, "Strings []"=w270) -> ()  [unwired: 2 in, 2 out]
                n166 = property on="Test Ring" class="Ring (strict)"("Visible"=TRUE) -> ()  [unwired: 2 in, 2 out]
                n167 = property on="Test Slider" class="Slide (strict)"("Visible"=FALSE) -> ()  [unwired: 2 in, 2 out]
              }
              frame Default {
                n168 = property on="Test Ring" class="Ring (strict)"("Visible"=FALSE) -> ()  [unwired: 2 in, 2 out]
                n169 = property on="Test Slider" class="Slide (strict)"("Visible"=FALSE) -> ()  [unwired: 2 in, 2 out]
              }
              frame "Brightness  **", "Color Level  **", "Compression  **", "FPS  **", "Sharpness  **" {
                n170 = call <vilib>:"NT Read Number.vi"("Name"=w282) -> ("Numeric"=w281:dbl)  [unwired: 9 in, 1 out]
                n171 = local write "Test Slider"(w281) -> ()
                n172 = property on="Test Slider" class="Slide (strict)"("Visible"=TRUE, "Scale.Maximum"=100.0 ("Scale.Range:Maximum")) -> ()  [unwired: 2 in, 2 out]
                n173 = property on="Test Ring" class="Ring (strict)"("Visible"=FALSE) -> ()  [unwired: 2 in, 2 out]
              }
            }
          }
        }
        n174 = property on="Progress" class="Clust (strict)"("Visible"=FALSE) -> ()  [unwired: 2 in, 2 out]
      }
      event "Test Name": Mouse Enter {
        # "Populate the ring with the list of tests"
        n175 = event-data() -> ()  [unwired: 1 in, 1 out]
        n176 = call <vilib>:"NT Read String Array.vi"("Name"="/TestMode/TestList") -> ("String Array"=w291:string[])  [unwired: 9 in, 1 out]
        n177 = Build Array (concatenate)("Select the test to run...", w291) -> (w290:string[])
        n178 = property on="Test Name" class="Ring (strict)"("Strings []"=w290) -> ()  [unwired: 2 in, 2 out]
      }
      event "Test Name": Value Change {
        w294 = FALSE ("Visible")
        # "Tell the robot the test name to run"
        n179 = event-data() -> ("NewVal"=w298:u16)  [unwired: 1 in]
        n180 = property on="Test Name" class="Ring (strict)"() -> ("Strings []"=w299:string[])  [unwired: 2 in, 2 out]
        n181 = local write "Progress"(T8 {"Test Progress"=0, "Test Progress Text"=""} ("Progress")) -> ()
        n182 = Index Array(array=w299, index=w298) -> (element=w297:string)
        n183 = call <vilib>:"NT Write String.vi"("String"=w297, "Name"="/TestMode/TestName") -> ()  [unwired: 9 in, 1 out]
        n184 = property on="Progress" class="Clust (strict)"("Visible"=TRUE) -> ()  [unwired: 2 in, 2 out]
        n185 = property on="Motor" class="Clust (strict)"("Visible"=w294) -> ()  [unwired: 2 in, 2 out]
        n186 = property on="Test Slider" class="Slide (strict)"("Visible"=w294) -> ()  [unwired: 2 in, 2 out]
        n187 = property on="On/Off" class="Bool (strict)"("Visible"=w294) -> ()  [unwired: 2 in, 2 out]
        n188 = property on="Rev/Fwd" class="Clust (strict)"("Visible"=w294) -> ()  [unwired: 2 in, 2 out]
        n189 = property on="Test Ring" class="Ring (strict)"("Visible"=w294) -> ()  [unwired: 2 in, 2 out]
      }
      event "Select Auto": Mouse Enter {
        # "Populate the combo box with the list of autonomous options"
        n190 = event-data() -> ()  [unwired: 1 in, 1 out]
        n191 = call <vilib>:"NT Read String Array.vi"("Name"="Auto List") -> ("String Array"=w301:string[])  [unwired: 9 in, 1 out]
        n192 = property on="Select Auto" class="CmbBox"("Strings[]"=w301) -> ()  [unwired: 2 in, 2 out]
      }
      event "Select Auto": Value Change {
        # "User modified the Auto Selection. Write to NT variable so robot knows."
        n193 = event-data() -> ("NewVal"=w305:string)  [unwired: 1 in]
        n194 = call <vilib>:"NT Write String.vi"("String"=w305, "Name"="Auto Selector") -> ()  [unwired: 9 in, 1 out]
      }
      event "Command Selection": Value Change {
        # "Get the params and show in table"
        n195 = event-data() -> ("NewVal"=w312:i32)  [unwired: 1 in]
        n196 = property on="Command Selection" class="MCListbox (strict)"() -> ("ItemNames"=w310:string[][])  [unwired: 2 in, 2 out]
        n197 = call <vilib>:"WPI_DashboardUpdate Command Params.vi"("NewVal"=w312, "Commands"=w310, "Param Tbl"=w311) -> ()  [unwired: 8 in, 1 out]
      }
      event "Execute Command": Value Change {
        # "Started one, Unique ID holds\nresponse"
        n198 = event-data() -> ()  [unwired: 1 in, 1 out]
        n199 = property on="Command Selection" class="MCListbox (strict)"() -> ("ItemNames"=w324:string[][])  [unwired: 2 in, 2 out]
        n200 = Index Array(array=w324, index (row)="Command Selection", index (col)=0) -> (element=w322:string)
        n201 = call <vilib>:"Invoke Commands.vi"("Command Params"="Command Params", "Function Name"=w322) -> ("Params"=w318:u8, "Started"=w317:bool)  [unwired: 7 in, 1 out]
        n202 = Array Subset(array="Command Params", length (row)=w318) -> (w319:string[][])  [unwired: 3 in]
        n203 = Select(t="Executing" ("Cmd Status"), s=w317, f="" ("Cmd Status")) -> (s? t:f=→"Cmd Status":string)
      }
      event "Command Selection": Double Click {
        n204 = event-data() -> ("Row"=w334:i32)  [unwired: 1 in]
        n205 = property on="Command Selection" class="MCListbox (strict)"() -> ("ItemNames"=w337:string[][])  [unwired: 2 in, 2 out]
        n206 = local read "Command Params"() -> (w332:string[][])
        n207 = Index Array(array=w337, index (row)=w334, index (col)=0) -> (element=w335:string)
        n208 = call <vilib>:"Invoke Commands.vi"("Command Params"=w332, "Function Name"=w335) -> ("Params"=w331:u8, "Started"=w326:bool)  [unwired: 7 in, 1 out]
        n209 = Array Subset(array=w332, length (row)=w331) -> (w330:string[][])  [unwired: 3 in]
        n210 = Select(t="Executing" ("Cmd Status"), s=w326, f="" ("Cmd Status")) -> (s? t:f=w327:string)
        n211 = local write "Cmd Status"(w327) -> ()
      }
      event "CheckList": Double Click {
        # "Shift clears all"
        # "Update symbols on the listbox"
        n212 = event-data() -> ("PlatMods.Shift"=w340:bool, "Row"=w342:i32)  [unwired: 1 in]
        n213 = case shown="True" w340 {
          tunnel: w342 -> [w346 _]
          tunnel: 1 -> [w345 _]
          frame False {
            n214 = property on="CheckList" class="LstBox (strict)"() -> ("Item Symbols"=w344:i32[])  [unwired: 2 in, 2 out]
            n215 = Replace Array Subset(array=w344, new element=w345, index=w346) -> (w343:i32[])
            n216 = property on="CheckList" class="LstBox (strict)"("Item Symbols"=w343) -> ()  [unwired: 2 in, 2 out]
          }
          frame True {
            w347 = 0 ("Top Row")
            n217 = property on="CheckList" class="LstBox (strict)"() -> ("Number of Rows"=w349:u32)  [unwired: 2 in, 2 out]
            n218 = Initialize Array(0, w349) -> (w348:i32[])
            n219 = property on="CheckList" class="LstBox (strict)"("Top Row"=w347, "Value"=w347, "Item Symbols"=w348) -> ()  [unwired: 2 in, 2 out]
          }
        }
      }
      event "CheckList": Key Down {
        # "Update symbols on the listbox\nLeft and right keys check and uncheck"
        n220 = event-data() -> ("VKey"=w354:T22)  [unwired: 1 in]
        n221 = case shown="\"Left\", \"Right\"" w354 {
          selector: w354 -> [w359 _]
          tunnel: eventvkey."Left" ("VKey") -> [w357 _]
          frame "Left", "Right" {
            n222 = Equal?(x=w357, y=w359) -> (x = y?=w358:bool)
            n223 = Select(t=0, s=w358, f=1) -> (s? t:f=w360:i32)
            n224 = property on="CheckList" class="LstBox (strict)"() -> ("Item Symbols"=w363:i32[])  [unwired: 2 in, 2 out]
            n225 = Replace Array Subset(array=w363, new element=w360, index="CheckList") -> (w362:i32[])
            n226 = property on="CheckList" class="LstBox (strict)"("Item Symbols"=w362) -> ()  [unwired: 2 in, 2 out]
          }
          frame Default {
          }
        }
      }
      event "DB Camera Config": Value Change {
        # "Show or hide the cluster of controls, store in ini file"
        n227 = event-data() -> ("NewVal"=w368:bool)  [unwired: 1 in]
        n228 = case shown="False" w368 {
          tunnel: w367 -> [w377 _]
          tunnel: [w370 w388] -> w366
          tunnel: w365 -> [w369 w388]
          frame False {
            w384 = "Camera"
            w387 = FALSE ("Visible")
            n229 = local read "Camera Settings"() -> (w376:T1)
            n230 = Index Array(array=w377) -> (element=w380:cluster{string[]})  [unwired: 1 in]
            n231 = Unbundle(w376) -> ("Frame Rate"=w375:i32, "Compression"=w374:i32, "Size"=w378:u16)
            n232 = Unbundle(w380) -> (w379:string[])
            n233 = Index Array(array=w379, index=w378) -> (element=w373:string)
            n234 = call-poly <vilib>:"Write Key.vi"("section"=w384, "value"=w373, "key"="Size", "refnum"=w369) -> ("refnum out"=w386:T20)  [unwired: 2 in, 5 out]
            n235 = call-poly <vilib>:"Write Key.vi"("section"=w384, "value"=w375, "key"="FrameRate", "refnum"=w386) -> ("refnum out"=w385:T20)  [unwired: 1 in, 6 out]
            n236 = property on="Camera Settings" class="Clust (strict)"("Visible"=w387) -> ()  [unwired: 2 in, 2 out]
            n237 = local write "DB Camera Config"(w387) -> ()
            n238 = call-poly <vilib>:"Write Key.vi"("section"=w384, "value"=w374, "key"="Compression", "refnum"=w385) -> ("refnum out"=w371:T20)  [unwired: 1 in, 6 out]
            n239 = call <vilib>:"Close Config Data.vi"("refnum"=w371) -> ("file path"=w372:path)  [unwired: 2 in, 8 out]
            n240 = call <vilib>:"Open Config Data.vi"("configuration file path"=w372) -> ("refnum"=w370:T20)  [unwired: 8 in, 2 out]
          }
          frame True {
            n241 = property on="Camera Settings" class="Clust (strict)"("Visible"=TRUE) -> ()  [unwired: 2 in, 2 out]
          }
        }
      }
      event "Camera Settings": Value Change {
        # "Update summary string when any elements of DB camera change"
        n242 = event-data() -> ("NewVal"=w402:T1)  [unwired: 1 in]
        n243 = Index Array(array=w398) -> (element=w397:cluster{string[]})  [unwired: 1 in]
        n244 = Unbundle(w402) -> ("Frame Rate"=w393:i32, "Compression"=w392:i32, "Size"=w395:u16)
        n245 = Unbundle(w397) -> (w396:string[])
        n246 = Index Array(array=w396, index=w395) -> (element=w394:string)
        n247 = Format Into String(format string="%s   %dfps   %d%%", w394, w393, w392) -> (resulting string=w399:string)  [unwired: 2 in, 1 out]
        n248 = Build Array(w399) -> (w400:string[])
        n249 = property on="DB Camera Config" class="Bool (strict)"("Strings [4]"=w400) -> ()  [unwired: 2 in, 2 out]
      }
      event "Motor.Enable": Value Change {
        # "When the test mode otor enable helper is set, update that\ntree row item's value"
        n250 = event-data() -> ("NewVal"=w409:bool)  [unwired: 1 in]
        n251 = Unbundle("Motor") -> ("Value"=w408:dbl)  [unwired: 1 out]
        n252 = Select(t=w408, s=w409, f=0.0) -> (s? t:f=w406:dbl)
        n253 = call <vilib>:"NT Write Number.vi"("Numeric"=w406, "Name"=w405) -> ()  [unwired: 9 in, 1 out]
      }
      event "Test Slider": Value Change {
        # "When the test mode slider helper is set, update that\ntree row item's value"
        n254 = event-data() -> ("NewVal"=w413:dbl)  [unwired: 1 in]
        n255 = call <vilib>:"NT Write Number.vi"("Numeric"=w413, "Name"=w414) -> ()  [unwired: 9 in, 1 out]
      }
      event "On/Off": Value Change {
        # "When the test mode on/off helper value is set, update that\ntree row item's value"
        n256 = event-data() -> ("NewVal"=w419:bool)  [unwired: 1 in]
        n257 = Boolean To (0,1)(Boolean=w419) -> (0, 1=w418:i16)
        n258 = call <vilib>:"NT Write Number.vi"("Numeric"=w418, "Name"=w417) -> ()  [unwired: 9 in, 1 out]
      }
      event "Rev/Fwd": Value Change {
        # "When the test mode helper value for relays is set, update that\ntree row item's value"
        n259 = event-data() -> ("NewVal.Forward"=w428:bool, "NewVal.Reverse"=w427:bool)  [unwired: 1 in]
        n260 = Boolean To (0,1)(Boolean=w428) -> (0, 1=w424:i16)
        n261 = Boolean To (0,1)(Boolean=w427) -> (0, 1=w426:i16)
        n262 = Negate(x=w426) -> (-x=w425:i16)
        n263 = Add(x=w424, y=w425) -> (x+y=w423:i16)
        n264 = call <vilib>:"NT Write Number.vi"("Numeric"=w423, "Name"=w422) -> ()  [unwired: 9 in, 1 out]
      }
      event "Test Ring": Value Change {
        # "When a test mode helper value is selected from the ring,\nset the tree item's variable to the string value"
        n265 = event-data() -> ("NewVal"=w433:u16)  [unwired: 1 in]
        n266 = property on="Test Ring" class="Ring (strict)"() -> ("Strings []"=w434:string[])  [unwired: 2 in, 2 out]
        n267 = Index Array(array=w434, index=w433) -> (element=w432:string)
        n268 = call <vilib>:"NT Write String.vi"("String"=w432, "Name"=w431) -> ()  [unwired: 9 in, 1 out]
      }
      event "Rec Mode": Value Change {
        # "Update globals for recording mode and path to read log from.\nClear when logging and let NetworkTables set path for vision to\nuse."
        n269 = event-data() -> ("NewVal"=w446:enum32{"Stop", "Record", "Playback"})  [unwired: 1 in]
        n270 = global write "WPI_DashboardLogging Global.vi" "Logging Filename"(path "") -> ()
        n271 = global write "WPI_DashboardLogging Global.vi" "Recording"(w446) -> ()
        n272 = case shown="\"Playback\"" w446 {
          tunnel: w445 -> [_ w448 w457]
          tunnel: [_ _ w456] -> w442
          tunnel: [_ _ w455] -> _
          tunnel: w440 -> [_ _ w453]
          tunnel: cluster{i32, i32} {-250, 170} -> [_ _ w452]
          tunnel: [_ _ T23 {"Image Size"=TRUE, "Image Type"=TRUE, "Pixel Value"=TRUE, "ROI Information"=TRUE, "Zoom Factor"=FALSE} ("Image Information Shown:All Elements")] -> w438
          tunnel: [_ _ TRUE ("Zoom Factor")] -> w437
          tunnel: w436 -> [_ _ w449]
          frame Default {
          }
          frame "Stop", "Record" {
            # "Place Window too"
            n273 = invoke class="VI" method="FP.Close"(reference=w448) -> (reference out=w447:refnum<vi>)  [unwired: 2 in, 2 out]
            n274 = invoke class="VI" method="Abort VI"(reference=w447) -> ()  [unwired: 2 in, 3 out]
          }
          frame "Playback" {
            n275 = call "Open Playback Panel.vi"("Offset"=w452, "DB VI Ref"=w453, "Playback in"=w457) -> ("Playback out"=w454:refnum<vi>)  [unwired: 8 in]
            n276 = register-events(w454, w449) -> (reference out=w456:refnum<event-registration>, error out=w455:errorcluster)  [unwired: 2 in]
          }
        }
        n277 = property on="Camera Image" class="ImageControl"("Image Information Shown"=w438, "Image Information Visible"=w437) -> ()  [unwired: 2 in, 2 out]
        n278 = call <vilib>:"WPI_DashboardNT Log FieldName Cache.vi"("Operation"=enum16{"Lookup/Add", "Index", "Clear"}."Clear") -> ()  [unwired: 8 in, 3 out]
      }
      event Panel Close {
        w459 = enum32{"Stop", "Record", "Playback"}."Stop" ("Rec Mode")
        # "Playback window has been closed, abort"
        n279 = event-data() -> ()  [unwired: 1 in, 4 out]
        n280 = local write "Rec Mode"(w459) -> ()
        n281 = global write "WPI_DashboardLogging Global.vi" "Recording"(w459) -> ()
      }
      event Panel Close {
        # "Abort playback window and ourself"
        n282 = event-data() -> ()  [unwired: 1 in, 4 out]
        n283 = invoke class="VI" method="FP.Close"(reference=w465) -> (reference out=w464:refnum<vi>)  [unwired: 2 in, 2 out]
        n284 = invoke class="VI" method="Abort VI"(reference=w464) -> (error out=w463:errorcluster)  [unwired: 2 in, 2 out]
        n285 = invoke class="VI" method="Abort VI"(error in=w463) -> ()  [unwired: 2 in, 3 out]
      }
      event User Event {
        n286 = event-data() -> ("IDs"=w473:cluster{"RPC field ID":u16, "Unique ID":u16}, "String"=w472:string)  [unwired: 1 in]
        n287 = Bundle("IDs"=w473, "String"=w472) -> (w471:T10)  [unwired: 1 in]
        n288 = call <vilib>:"Retrieve RPC Response.vi"("RPC Response"=w471) -> ("Output"=w468:string[][])  [unwired: 10 in]
        n289 = Build Array (concatenate)(w466, w468) -> (w467:string[][])
        n290 = local write "Command Params"(w467) -> ()
        n291 = local write "Cmd Status"("" ("Cmd Status")) -> ()
      }
      event "Vision": Value Change {
        # "Enable/Disable Compression slider.\nHW USB is hard-coded into the camera"
        n292 = event-data() -> ("NewVal"=w480:u16)  [unwired: 1 in]
        n293 = Equal?(x=w480, y=u32 2 ("milliseconds to wait")) -> (x = y?=w478:bool)
        n294 = Select(t=T24."Disabled and Grayed Out" ("Disabled"), s=w478, f=T24."Enabled" ("Disabled")) -> (s? t:f=w475:T24)
        n295 = property on="Compression" class="Slide (strict)"("DisabledEnum"=w475) -> ()  [unwired: 2 in, 2 out]
      }
      event "Tree": Double Click {
        n296 = event-data() -> ("PlatMods"=w485:T27, "Tag"=w484:string)  [unwired: 1 in]
        n297 = Unbundle(w485) -> ("Shift"=w483:bool)  [unwired: 4 out]
        n298 = Not(x=w483) -> (.not. x?=w482:bool)
        n299 = call <vilib>:"NT Update Persistence.vi"("Persistence"=w482, "Name"=w484) -> ()  [unwired: 9 in, 1 out]
      }
    }
  }
  n300 = while {
    tunnel: w51 -> [w489]
    i -> [w492]
    stop <- FALSE stop-if-true
    n301 = Wait (ms)(milliseconds to wait=u32 100) -> ()  [unwired: 1 out]
    n302 = case shown="\"Playback\"" "Rec Mode" {
      tunnel: w492 -> [_ _ w507]
      tunnel: [u32 2829099 ("Base Color") u32 11141120 ("Target Color") w496] -> w488
      frame "Stop", Default {
        # "Reset the color, extra updates don't cost much"
      }
      frame "Record" {
      }
      frame "Playback" {
        # "Playback"
        n303 = Quotient & Remainder(x=w507, y=u32 50 ("milliseconds to wait")) -> (x-y*floor(x/y)=w503:u32)  [unwired: 1 out]
        n304 = Divide(x=w503, y=u32 50 ("milliseconds to wait")) -> (x/y=w500:dbl)
        n305 = Multiply(x=6.283185307179586, y=w500) -> (x*y=w505:dbl)
        n306 = Sine(x=w505) -> (sin(x)=w504:dbl)
        n307 = Absolute Value(x=w504) -> (abs(x)=w497:dbl)
        n308 = call "Interpolate RGB Color.vi"("Proportion"=w497, "Target Color"=u32 30976, "Base Color"=u32 2829099) -> ("Result Color"=w496:u32)  [unwired: 8 in]
      }
    }
    n309 = property class="Pane"(reference=w489, "PaneColor"=w488) -> ()  [unwired: 1 in, 2 out]
  }
  n310 = local write "Dashboard Tab"(T2."Drive" ("Dashboard Tab")) -> ()
  n311 = property on="On/Off" class="Bool (strict)"("Visible"=w19) -> ()  [unwired: 2 in, 2 out]
  n312 = property on="Motor" class="Clust (strict)"("Visible"=w19) -> ()  [unwired: 2 in, 2 out]
  n313 = property on="Progress" class="Clust (strict)"("Visible"=w19) -> ()  [unwired: 2 in, 2 out]
  n314 = property on="Test Ring" class="Ring (strict)"("Visible"=w19) -> ()  [unwired: 2 in, 2 out]
  n315 = property on="Rev/Fwd" class="Clust (strict)"("Visible"=w19) -> ()  [unwired: 2 in, 2 out]
  n316 = property on="Camera Settings" class="Clust (strict)"("Visible"=w19) -> ()  [unwired: 2 in, 2 out]
  n317 = while {
    tunnel: u16 1741 ("timeout ms (25000)") -> [w509]
    stop <- FALSE stop-if-true
    n318 = TCP Create Listener(10:w509) -> (0:w508:errorcluster, 3:w510:refnum<k5>)  [unwired: 4 in, 1 out]
    n319 = case shown="No Error" w508 {
      selector: w508 -> [w512 _]
      tunnel: w510 -> [w513 _]
      frame No Error {
        n320 = while {
          tunnel: w513 -> [w516]
          tunnel: w512 -> [w515]
          stop <- FALSE stop-if-true
          n321 = TCP Wait On Listener(8:w515, 11:w516) -> (0:w517:errorcluster, 4:w518:refnum<k5>)  [unwired: 2 in, 3 out]
          n322 = local write "TCP"(w518) -> ()
          n323 = case shown="No Error" w517 {
            frame No Error {
            }
            frame Error {
              n324 = Wait (ms)(milliseconds to wait=u32 1000) -> ()  [unwired: 1 out]
            }
          }
        }
      }
      frame Error {
        n325 = Wait (ms)(milliseconds to wait=u32 1000) -> ()  [unwired: 1 out]
      }
    }
  }
  n326 = local write "DB Camera Config"(w19) -> ()
  n327 = local write "Command Params"(string[][] [] ("Command Params")) -> ()
  n328 = global write "WPI_DashboardLogging Global.vi" "Recording"(w45) -> ()
  n329 = local write "Command Selection"(u16 0 ("milliseconds to wait")) -> ()
  n330 = local write "Rec Mode"(w45) -> ()
  n331 = call "IMAQ Create"("Image Name"="Dashboard Image", "Image Type"=w65) -> ("New Image"=w63:T7, "error out"=w62:errorcluster)  [unwired: 2 in, 1 out]
  n332 = while {
    tunnel: w63 -> [w529]
    tunnel: w62 -> [_]
    tunnel: [w530] -> _
    i -> [w530]
    stop <- FALSE stop-if-true
    # "Optionally read the DB image,\nlog, or retrieve images from a\nlogged match"
    n333 = local read "Rec Mode"() -> (w524:enum32{"Stop", "Record", "Playback"})
    n334 = local read "Camera IP"() -> (w522:string)
    n335 = call <vilib>:"WPI_CameraRead MJPG for Dashboard.vi"("Camera Settings"="Camera Settings", "Rec Mode"=w524, "Camera IP"=w522, "Camera Mode"="Vision", "Refnum in"=w529) -> ("Active"=w527:bool, "Refnum out"=w528:T7, "FPS"=w526:dbl, "Bandwidth (Mbps)"=w521:dbl)  [unwired: 3 in]
    "Mbps" <- w521
    n336 = case shown="False" w527 {
      tunnel: w528 -> [_ w539]
      tunnel: w521 -> [_ w538]
      tunnel: w526 -> [_ w536]
      frame False {
        w532 = u32 1985280 ("Color Box")
        # "Sleep for 500ms"
        n337 = Bundle("Color Box"=w532, "Color Box"=w532) -> (w534:cluster{"Color Box":u32, "Color Box":u32})  [unwired: 1 out]
        n338 = Build Array(w534) -> (w533:cluster{"Color Box":u32, "Color Box":u32}[])
        n339 = property on="Mbps LED" class="Bool (strict)"("Colors [4]"=w533) -> ()  [unwired: 2 in, 2 out]
        n340 = Wait Until Next ms Multiple(millisecond multiple=u32 500) -> ()  [unwired: 1 out]
      }
      frame True {
        # "Here is where you would annotate,\npossibly process, and display the image"
        # "Update Mbps LED"
        n341 = call "IMAQ Clear Overlay"("Image"=w539) -> ("error out"=w543:errorcluster, "Image Out"=→"Camera Image":T7)  [unwired: 2 in, 7 out]
        n342 = case shown="Default" w538 {
          tunnel: [u32 6618880 ("Color Box") u32 16776722 ("Color Box") u32 16716800 ("Color Box")] -> w540
          frame Default {
          }
          frame 4, 5 {
          }
          frame 6.. {
          }
        }
        n343 = Unbundle By Name(w543) -> ("status"=w544:bool)
        n344 = Bundle("Color Box"=w540, "Color Box"=w540) -> (w542:cluster{"Color Box":u32, "Color Box":u32})  [unwired: 1 out]
        n345 = property on="Image Message" class="Str"("Visible"=w544) -> ()  [unwired: 2 in, 2 out]
        n346 = Build Array(w542) -> (w541:cluster{"Color Box":u32, "Color Box":u32}[])
        n347 = property on="Mbps LED" class="Bool (strict)"("Colors [4]"=w541) -> ()  [unwired: 2 in, 2 out]
        "fps" <- w536
      }
    }
  }
  n348 = call "IMAQ Create"("Image Name"="Dashboard Image", "Image Type"=w4) -> ("New Image"=w2:T7, "error out"=w1:errorcluster)  [unwired: 2 in, 1 out]
  n349 = while {
    tunnel: w2 -> [w556]
    tunnel: w1 -> [_]
    tunnel: [w557] -> _
    i -> [w557]
    stop <- FALSE stop-if-true
    # "Optionally read the DB image,\nlog, or retrieve images from a\nlogged match"
    n350 = local read "Rec Mode 2"() -> (w551:enum32{"Stop", "Record", "Playback"})
    n351 = local read "Camera IP 2"() -> (w549:string)
    n352 = call <vilib>:"WPI_CameraRead MJPG for Dashboard.vi"("Camera Settings"="Camera Settings 2", "Rec Mode"=w551, "Camera IP"=w549, "Camera Mode"="Vision 2", "Refnum in"=w556) -> ("Active"=w554:bool, "Refnum out"=w555:T7, "FPS"=w553:dbl, "Bandwidth (Mbps)"=w548:dbl)  [unwired: 3 in]
    "Mbps 2" <- w548
    n353 = case shown="True" w554 {
      tunnel: w555 -> [_ w562]
      tunnel: w548 -> [_ _]
      tunnel: w553 -> [_ w560]
      frame False {
        # "Sleep for 500ms"
        n354 = Wait Until Next ms Multiple(millisecond multiple=u32 500) -> ()  [unwired: 1 out]
      }
      frame True {
        # "Here is where you would annotate,\npossibly process, and display the image"
        n355 = call "IMAQ Clear Overlay"("Image"=w562) -> ("error out"=w563:errorcluster, "Image Out"=→"Camera Image 2":T7)  [unwired: 2 in, 7 out]
        n356 = Unbundle By Name(w563) -> ()  [unwired: 1 out]
        "fps 2" <- w560
      }
    }
  }
